vi "DPDDdll.vi"(8 "error in (no error)":errorcluster, 9 "z":dbl[](array[numeric]), 10 "D":dbl, 11 "t":dbl) -> (0 "error out":errorcluster, 3 "dPdD out":dbl)   [LabVIEW 2021]
doc: "subroutine DPDD (t,D,z,dpdD)\n\nCompute partial derivative of pressure w.r.t. density at constant\ntemperature as a function of temperature, density, and composition\n\nINPUTS:\nt --temperature [K]\nD --molar density [mol/L]\nz --composition [array of mol frac]\n\nOUTPUTS:\ndpdD --dP/drho [kPa-L/mol]"
uses:
  REFPROP.dll
panel:
  # "REFPROP-DPDDdll.vi"
  # "void  DPDDdll(double *t, double *D, double *z, double *dpdD);"
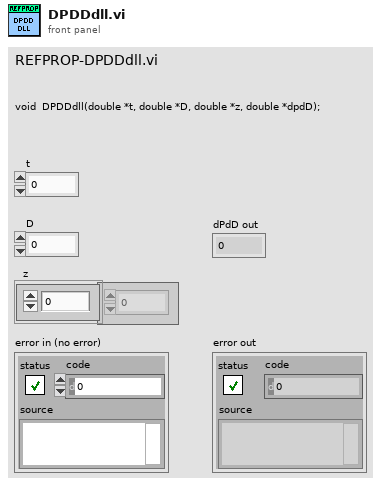
[diagram p1: front panel]
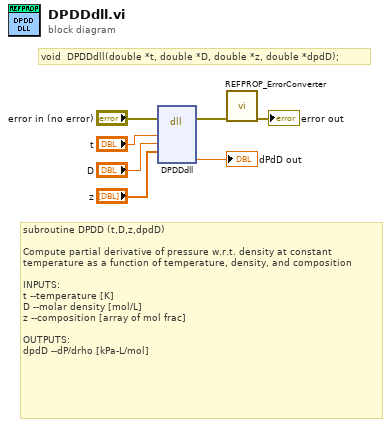
[diagram p0: block diagram]
diagram:
  # "void  DPDDdll(double *t, double *D, double *z, double *dpdD);"
  # "subroutine DPDD (t,D,z,dpdD)\n\nCompute partial derivative of pressure w.r.t. density at constant\ntemperature as a function of temperature, density, and composition\n\nINPUTS:\nt --temperature [K]\nD --molar density [mol/L]\nz --composition [array of mol frac]\n\nOUTPUTS:\ndpdD --dP/drho [kPa-L/mol]"
  n1 = dll-call lib="C:/Users/lauria/OneDrive - National Institute of Standards and Technology (NIST)/LabVIEW Projects/7 REFPROP/REFPROP-wrappers-master/REFPROP-wrappers-master/wrappers/Labview/REFPROP/REFPROP.*" fn="DPDDdll"(error in="error in (no error)", "t"="t", "D"="D", "z"="z") -> (error out=w3:errorcluster, "dpdD"=→"dPdD out":dbl)  [unwired: 7 in, 1 out]
  n2 = call "REFPROP_ErrorConverter.vi"("error in (no error)"=w3) -> ("error out"=→"error out":errorcluster)  [unwired: 10 in]
